vi "Z6_Beamline_Chief.constructor.vi"(0 "name":string, 2 "data in":string, 5 "error in":errorcluster) -> (14 "i ref out":refnum<vi>, 16 "data out":string, 19 "error out":errorcluster)   [LabVIEW 2014, in "Z6_Beamline_Chief.lvlib"]
doc: "This class is forseen to inspect the PHELIX beamline and to select the mode. Additional several settings can be chosen.\n\nThis class is part of the PHELIX user layer.\n\nauthor: Stefan Götte, GSI\n\nLicense Agreement for this software:\n\nCopyright (C)\nGesellschaft für Schwerionenforschung, GSI\nPlanckstr. 1\n64291 Darmstadt\nGermany\n\nContact: D.Beck@gsi.de \n\nThis program is free software; you can redistribute it and/or modify it under the terms of the \nGNU General Public License as published by the Free Software Foundation; either version 2 of \nthe license, or (at your option) any later version.\n\nThis program is distributed in the hope that it will be useful, but WITHOUT ANY WARRANTY; \nwithout even the implied warranty of MERCHANTABILITY or FITNESS FOR A PARTICULAR PURPOSE. See the GNU General License for more details (http://www.gnu.org).\n\nGesellschaft für Schwerionenforschung, GSI\nPlanckstr. 1, 64291 Darmstadt, Germany\nFor all questions and ideas contact: M.Richter@gsi.de, H.Brand@gsi.de or D.Beck@gsi.de.\nLast update: 16-JUN-2004"
uses:
  Z6_Beamline_Chief.lvlib
  CSCore/CSSystem/CSSystemLib/CSSystemLib.lvlib
  Z6_Beamline/Z6_Beamline.lvlib
  CSCore/CSObj/CSObj.lvlib
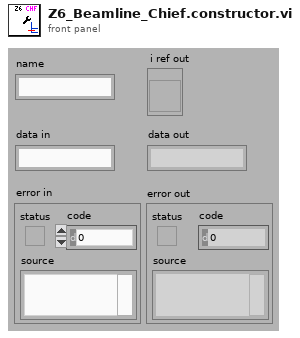
[diagram p1: front panel]
types:
  T1 = enum16{"SetAttribute", "GetAttribute", "CreateAttribute", "DestroyAttribute", "DestroyAllAtributes"}
  T2 = typedef "Z6_Beamline_Chief.lvlib/Z6_Beamline_Chief.i attribute.ctl" = cluster{"R2S Service ID":i32}
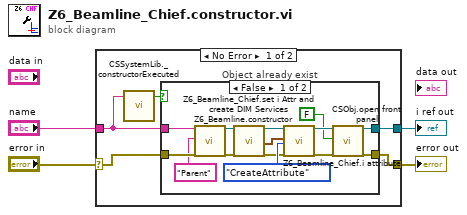
[diagram p0: block diagram]
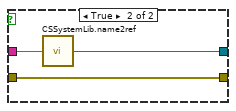
[diagram p2: hidden frame]
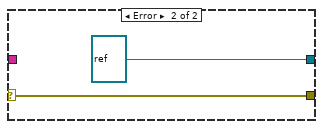
[diagram p3: hidden frame]
diagram:
  n1 = case shown="No Error" "error in" {
    selector: "error in" -> [w5 w28]
    tunnel: "name" -> [w6 _]
    tunnel: [w8 w28] -> w3
    tunnel: [w7 refnum<vi> refnum ("i ref out")] -> w2
    frame No Error {
      n2 = call "CSSystemLib._constructorExecuted.vi"("name"=w6) -> ("constructor executed?"=w9:bool)  [unwired: 18 in]
      n3 = case "Object already exist" shown="False" w9 {
        tunnel: w6 -> [w22 w26]
        tunnel: [w12 w25] -> w8
        tunnel: w5 -> [w16 w25]
        tunnel: [w13 w24] -> w7
        frame False {
          n4 = call "Z6_Beamline.constructor.vi"("name"=w22, "data in"="Parent", "error in"=w16) -> ("i ref out"=w17:refnum<vi>, "error out"=w18:errorcluster)  [unwired: 14 in, 1 out]
          n5 = call "Z6_Beamline_Chief.set i Attr and create DIM Services.vi"("Refnum in"=w17, "error in"=w18) -> ("i ref out"=w21:refnum<vi>, "i Attr"=w19:T2, "error out"=w20:errorcluster)  [unwired: 15 in]
          n6 = call "Z6_Beamline_Chief.i attribute.vi"("VI Refnum"=w21, "CLASS.i attribute"=w19, "Action"=T1."CreateAttribute", "error in (no error)"=w20) -> ("VI Refnum out"=w15:refnum<vi>, "error out"=w14:errorcluster)  [unwired: 13 in, 1 out]
          n7 = call "CSObj.open front panel.vi"("i ref in"=w15, "frontPanelOpen"=FALSE, "error in (no error)"=w14) -> ("i ref out"=w13:refnum<vi>, "error out"=w12:errorcluster)  [unwired: 15 in]
        }
        frame True {
          n8 = call "CSSystemLib.name2ref.vi"("name"=w26) -> ("obj refnum"=w24:refnum<vi>)
        }
      }
    }
    frame Error {
    }
  }
  "i ref out" <- w2
  "error out" <- w3
